vi "Power_spectrum_Autocorrelation.vi"(5 "Spectrum input array":dbl[](array[numeric]) format="%.2f", 7 "Time Trace":T2, 8 "Cluster in":T3={"Colour"=0, "Inst type"=enum."Pitot-static tube", "Inst name"="Manometer voltage", "Symbol"="U", "Code name"="", "Extra Info"="U", "Inst Array"=enum."PWA", "Extra Titles"=[], "Extra Values"=[], "U"=0.0, "u^2"=0.0, "u^3"=0.0, "u^4"=0.0, "Skew_u"=0.0, "Kurt_u"=0.0, "Sd Error in Mean"=0.0, "% u'/U"=0.0, "X"=0.0, "Y"=0.0, "Z"=0.0, "Timescale integral to 25%"=0.0, "Sd Error in Variance"=0.0, "Calib File"=path "", "Calib Constants"=[], "Output Position"=FALSE, "Full Stats"=FALSE, "Av Sampling Rate"=0.0, "Av No of Samples"=0.0, "Total Meas Time (s)"=0.0, "ADAM Ch Name"=""} {"Sd Error in Variance" format="%.2f"; "Skew_u" format="%.2f"; "% u'/U" format="%.2f"; "Sd Error in Mean" format="%.2f"; "Kurt_u" format="%.2f"; "u^4" format="%.2f"; "u^3" format="%.2f"; "U" format="%.2f"; "u^2" format="%.2f"}) -> (0 "Spectrum output array":dbl[](array[numeric]) format="%.2f", 1 "Autocorrelation":T1, 2 "Spectra":T1, 3 "Cluster Out":T3={"Colour"=0, "Inst type"=enum."Pitot-static tube", "Inst name"="Manometer voltage", "Symbol"="U", "Code name"="", "Extra Info"="U", "Inst Array"=enum."PWA", "Extra Titles"=[], "Extra Values"=[], "U"=0.0, "u^2"=0.0, "u^3"=0.0, "u^4"=0.0, "Skew_u"=0.0, "Kurt_u"=0.0, "Sd Error in Mean"=0.0, "% u'/U"=0.0, "X"=0.0, "Y"=0.0, "Z"=0.0, "Timescale integral to 25%"=0.0, "Sd Error in Variance"=0.0, "Calib File"=path "", "Calib Constants"=[], "Output Position"=FALSE, "Full Stats"=FALSE, "Av Sampling Rate"=0.0, "Av No of Samples"=0.0, "Total Meas Time (s)"=0.0, "ADAM Ch Name"=""} {"Sd Error in Variance" format="%.2f"; "Skew_u" format="%.2f"; "% u'/U" format="%.2f"; "Sd Error in Mean" format="%.2f"; "Kurt_u" format="%.2f"; "u^4" format="%.2f"; "u^3" format="%.2f"; "U" format="%.2f"; "u^2" format="%.2f"})   [LabVIEW 2012]
uses:
  Controls/Analysis_info_cluster.ctl
  Controls/Inst_type.ctl
  Controls/Instrument_Array.ctl
  Controls/Time_Trace_Cluster.ctl
  Controls/XY_Plot_Cluster.ctl
  Globals/Meas_global.vi
  <vilib>/gmath/NI_Gmath.lvlib
panel:
  out "Numeric":dbl
  out "size(s)":i32
  out "XY Graph 2":cluster{dbl[], dbl[]}(graph)
  in  "method":i32(ring) items=["nearest", "linear", "spline", "cubic Hermite", "Lagrange"]
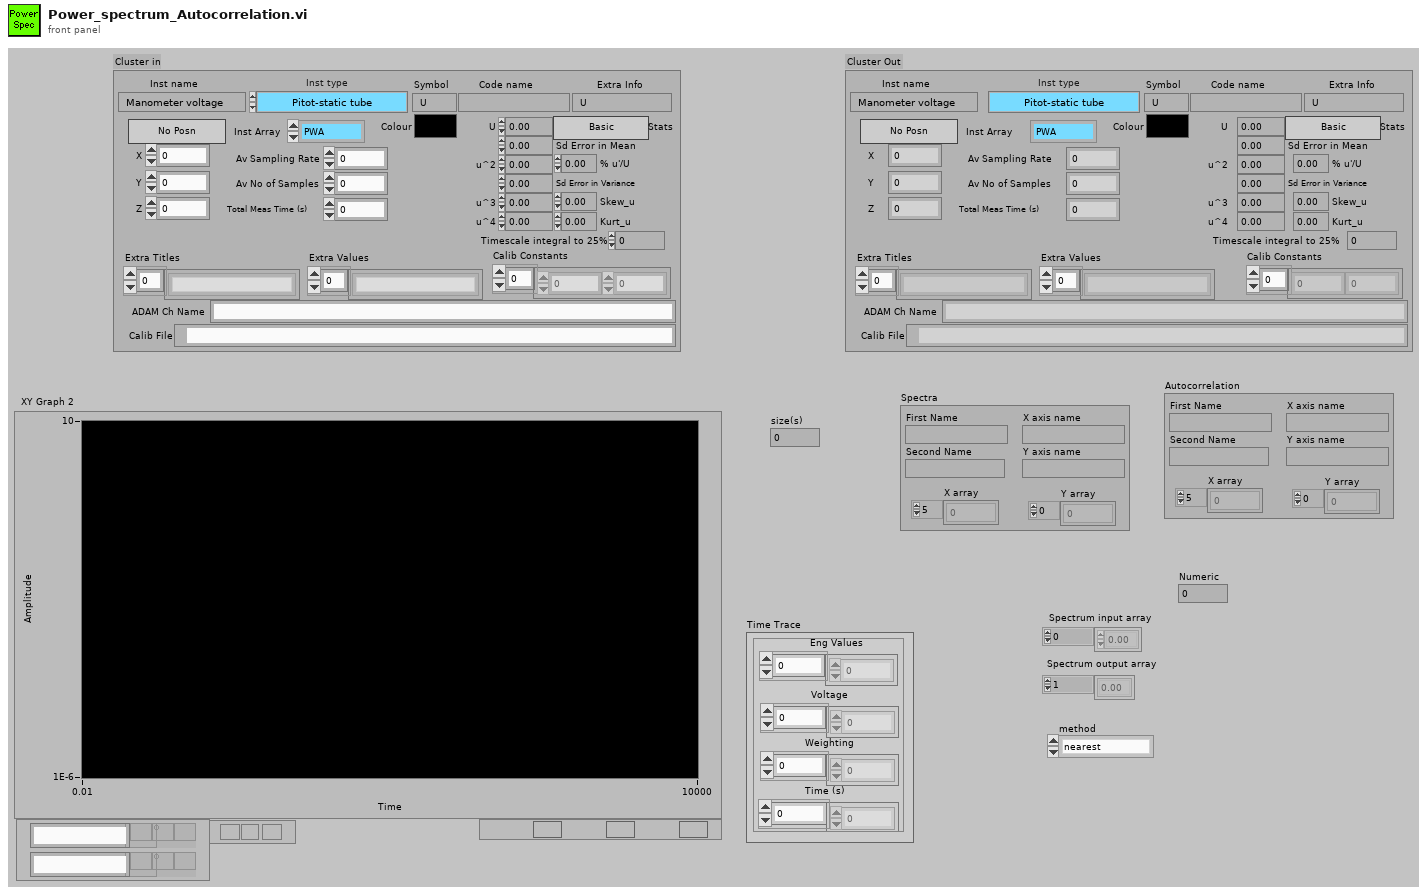
[diagram p1: front panel]
types:
  T1 = typedef "XY_Plot_Cluster.ctl" = cluster{"First Name":string, "Second Name":string, "X axis name":string, "Y axis name":string, "X array":dbl[], "Y array":dbl[]}
  T2 = typedef "Time_Trace_Cluster.ctl" = cluster{"Weighting":dbl[], "Time (s)":dbl[], "Voltage":dbl[], "Eng Values":dbl[]}
  T3 = typedef "Analysis_info_cluster.ctl" = cluster{"Colour":u32, "Inst type":T4, "Inst name":string, "Symbol":string, "Code name":string, "Extra Info":string, "Inst Array":T5, "Extra Titles":string[], "Extra Values":string[], "U":dbl, "u^2":dbl, "u^3":dbl, "u^4":dbl, "Skew_u":dbl, "Kurt_u":dbl, "Sd Error in Mean":dbl, "% u'/U":dbl, "X":dbl, "Y":dbl, "Z":dbl, "Timescale integral to 25%":dbl, "Sd Error in Variance":dbl, "Calib File":path, "Calib Constants":dbl[], "Output Position":bool, "Full Stats":bool, "Av Sampling Rate":dbl, "Av No of Samples":dbl, "Total Meas Time (s)":dbl, "ADAM Ch Name":string}
  T4 = typedef "Inst_type.ctl" = enum16{"Propeller anemometer", "Raw voltage", "Pressure Transducer", "Pitot-static tube", "Preston tube", "Hot wire", "Cross wire 1", "Cross wire 2", "Generic Linear", "Generic Polynomial", "Generic BackPoly", "Fast FID", "Thermocouple", "Cold wire", "Pulsed Wire", "LDA Vel", "LDA Tran time", "LDA Arr time"}
  T5 = typedef "Instrument_Array.ctl" = enum16{"PWA", "LDA", "Analogue"}
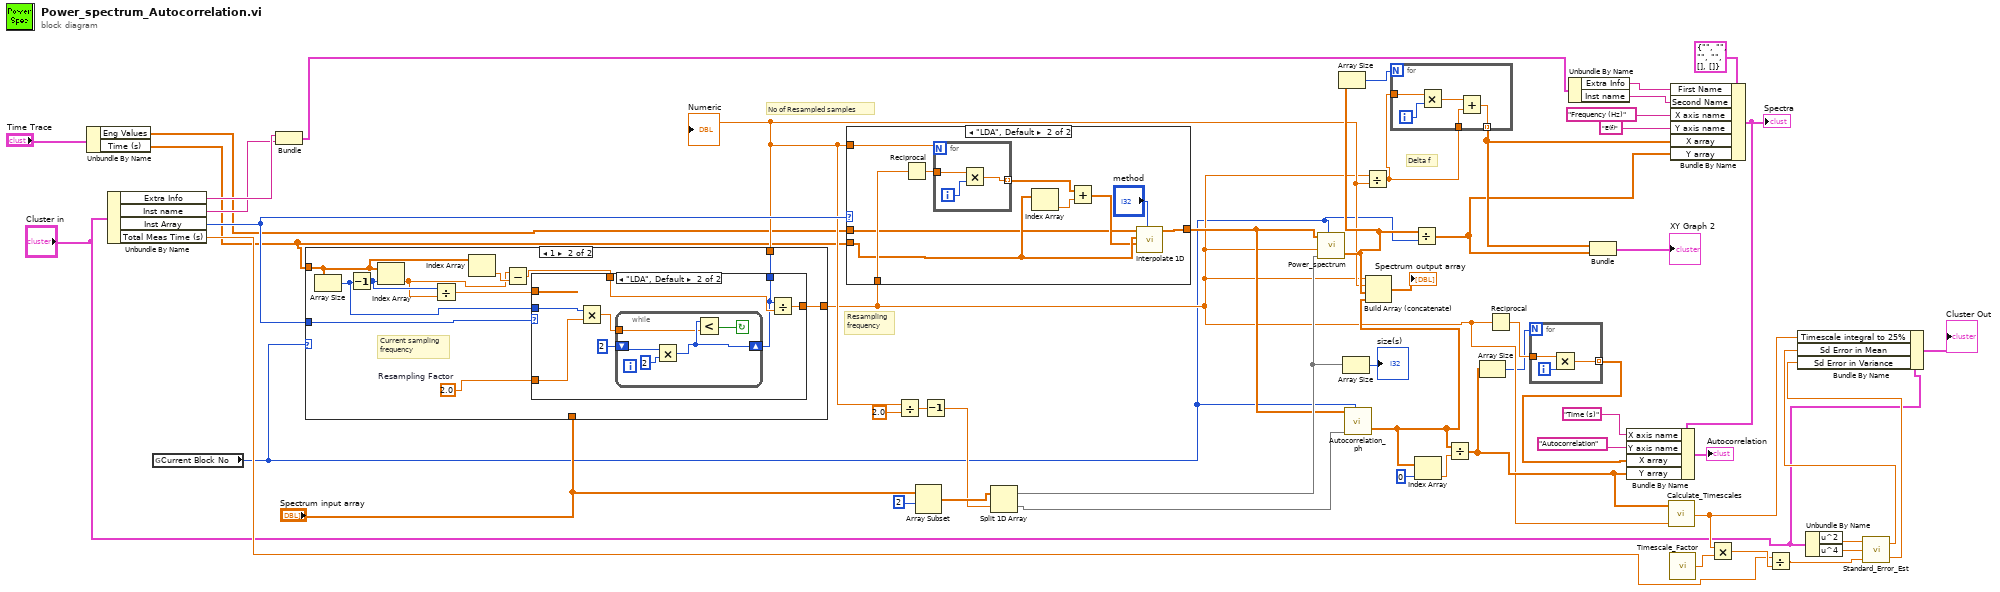
[diagram p0: block diagram]
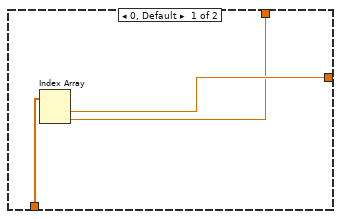
[diagram p2: hidden frame]
diagram:
  # "No of Resampled samples"
  # "Resampling\nfrequency"
  # "Delta f"
  n1 = Unbundle By Name("Time Trace") -> ("Eng Values"=w7:dbl[], "Time (s)"=w3:dbl[])
  n2 = Unbundle By Name("Cluster in") -> ("Extra Info"=w48:string, "Inst name"=w46:string, "Inst Array"=w52:T5, "Total Meas Time (s)"=w9:dbl)
  n3 = global read "Meas_global.vi" "Current Block No"() -> (w1:i32)
  n4 = Bundle("Extra Info"=w48, "Inst name"=w46) -> (w47:cluster{"Extra Info":string, "Inst name":string})  [unwired: 1 in]
  n5 = case shown="1" w1 {
    tunnel: w3 -> [_ w61]
    tunnel: [w56 w66] -> w19
    tunnel: "Spectrum input array" -> [w57 _]
    tunnel: w52 -> [_ w67]
    tunnel: [w55 w64] -> w35
    frame 0, Default {
      n6 = Index Array(array=w57) -> (element #1=w56:dbl, element #2=w55:dbl)  [unwired: 2 in]
    }
    frame 1 {
      w62 = 2.0  # Resampling Factor
      # "Current sampling\nfrequency"
      n7 = Array Size(array=w61) -> (size(s)=w63:i32)
      n8 = Decrement(x=w63) -> (x-1=w65:i32)
      n9 = Index Array(array=w61, index=w65) -> (element=w58:dbl)
      n10 = Divide(x=w65, y=w58) -> (x/y=w68:dbl)
      n11 = Index Array(array=w61) -> (element=w60:dbl)  [unwired: 1 in]
      n12 = Subtract(x=w58, y=w60) -> (x-y=w59:dbl)
      n13 = case shown="\"LDA\", Default" w67 {
        tunnel: w68 -> [w70 _]
        tunnel: w59 -> [_ w77]
        tunnel: [w70 w76] -> w66
        tunnel: w63 -> [w69 w74]
        tunnel: [w69 w73] -> w64
        tunnel: w62 -> [_ w72]
        frame "Analogue" {
        }
        frame "LDA", Default {
          n14 = Multiply(x=w74, y=w72) -> (x*y=w75:dbl)
          n15 = while {
            shift-right: [w80] -> w73
            shift-left: 2 -> [w82]
            tunnel: w75 -> [w78]
            stop <- w79 continue-if-true
            n16 = Multiply(x=w82, y=2) -> (x*y=w80:i32)
            n17 = Less?(x=w80, y=w78) -> (x < y?=w79:bool)
          }
          n18 = Divide(x=w73, y=w77) -> (x/y=w76:dbl)
        }
      }
    }
  }
  "Numeric" <- w35
  n19 = case shown="\"LDA\", Default" w52 {
    tunnel: w7 -> [w83 w84]
    tunnel: w3 -> [_ w88]
    tunnel: [w83 w92] -> w30
    tunnel: w35 -> [_ w91]
    tunnel: w19 -> [_ w89]
    frame "Analogue" {
    }
    frame "LDA", Default {
      n20 = Reciprocal(x=w89) -> (1/x=w90:dbl)
      n21 = for {
        N: w91 -> [_]
        tunnel: w90 -> [w96]
        tunnel: [w94] -> w86 mode=indexing
        i -> [w95]
        n22 = Multiply(x=w96, y=w95) -> (x*y=w94:dbl)
      }
      n23 = Index Array(array=w88) -> (element=w87:dbl)  [unwired: 1 in]
      n24 = Add(x=w86, y=w87) -> (x+y=w85:dbl[])
      n25 = call <vilib>:"Interpolate 1D.vi"("method"="method", "xi"=w85, "X"=w88, "Y"=w84) -> ("yi"=w92:dbl[])  [unwired: 2 in, 5 out]
    }
  }
  n26 = Divide(x=w35, y=2.0) -> (x/y=w33:dbl)
  n27 = Array Subset(array="Spectrum input array", index=2) -> (w36:dbl[])  [unwired: 1 in]
  n28 = Decrement(x=w33) -> (x-1=w32:dbl)
  n29 = Split 1D Array(array=w36, index=w32) -> (first subarray=w31:dbl[], second subarray=w29:dbl[])
  n30 = call "Power_spectrum.vi"("U"=w30, "Sampling frequency"=w19, "Spectrum input array"=w31, "Block No"=w1) -> ("Spectrum output array"=w40:dbl[])  [unwired: 2 in]
  n31 = Array Size(array=w40) -> (size(s)=w50:i32)
  n32 = Array Size(array=w31) -> (size(s)=→"size(s)":i32)
  n33 = call "Autocorrelation_ph.vi"("X"=w30, "Autocorrelation of X"=w29, "Block No"=w1) -> ("Autocorrelation of X"=w26:dbl[])  [unwired: 2 in, 1 out]
  n34 = Divide(x=w19, y=w35) -> (x/y=w51:dbl)
  n35 = Build Array (concatenate)(w19, w35, w40, w26) -> (→"Spectrum output array":dbl[])
  n36 = for {
    N: w50 -> [_]
    tunnel: w51 -> [w101]
    tunnel: w51 -> [w98]
    tunnel: [w97] -> w41 mode=indexing
    i -> [w100]
    n37 = Multiply(x=w101, y=w100) -> (x*y=w99:dbl)
    n38 = Add(x=w99, y=w98) -> (x+y=w97:dbl)
  }
  n39 = Divide(x=w40, y=w1) -> (x/y=w39:dbl[])
  n40 = Index Array(array=w26, index=0 ("Index")) -> (element=w27:dbl)
  n41 = Divide(x=w26, y=w27) -> (x/y=w21:dbl[])
  n42 = Array Size(array=w21) -> (size(s)=w18:i32)
  n43 = Reciprocal(x=w19) -> (1/x=w23:dbl)
  n44 = for {
    N: w18 -> [_]
    tunnel: w23 -> [w103]
    tunnel: [w102] -> w22 mode=indexing
    i -> [w104]
    n45 = Multiply(x=w103, y=w104) -> (x*y=w102:dbl)
  }
  n46 = Unbundle By Name(w47) -> ("Extra Info"=w45:string, "Inst name"=w44:string)
  n47 = Bundle(w41, w39) -> (→"XY Graph 2":cluster{dbl[], dbl[]})  [unwired: 1 in]
  n48 = call "Calculate_Timescales.vi"("Sampling Frequency (Hz)"=w19, "Autocorrelation"=w21) -> ("Time Scale estimate (s)"=w16:dbl)  [unwired: 1 in]
  n49 = call "Timescale_Factor.vi"() -> ("Factor to scale timescale by"=w17:dbl)
  n50 = Bundle By Name(cluster=T1 {"First Name"="", "Second Name"="", "X axis name"="", "Y axis name"="", "X array"=[], "Y array"=[]} ("element"), "First Name"=w45, "Second Name"=w44, "X axis name"="Frequency (Hz)", "Y axis name"="E(f)", "X array"=w41, "Y array"=w39) -> (w5:T1)
  "Spectra" <- w5
  n51 = Bundle By Name(cluster=w5, "X axis name"="Time (s)", "Y axis name"="Autocorrelation", "X array"=w22, "Y array"=w21) -> (→"Autocorrelation":T1)
  n52 = Multiply(x=w16, y=w17) -> (x*y=w13:dbl)
  n53 = Divide(x=w9, y=w13) -> (x/y=w12:dbl)
  n54 = Unbundle By Name("Cluster in") -> ("u^2"=w15:dbl, "u^4"=w14:dbl)
  n55 = call "Standard_Error_Est.vi"("N"=w12, "4th order moment u^4"=w14, "2nd order moment u^2"=w15) -> ("Standard error in variance"=w10:dbl, "Standard error in Mean"=w11:dbl)
  n56 = Bundle By Name(cluster="Cluster in", "Timescale integral to 25%"=w16, "Sd Error in Mean"=w11, "Sd Error in Variance"=w10) -> (→"Cluster Out":T3)
